vi "DeviceTestPanelGetTimeSeriesRequest_Create.vi"(7 "Header":T2, 8 "error in (no error)":errorcluster, 9 "DeviceTestPanelGetTimeSeriesRequest":T1, 10 "SendTo":string, 11 "ReplyTo":string) -> (0 "error out":errorcluster, 3 "Message":T4)   [LabVIEW 2017]
uses:
  <vilib>/addons/InsightCM/MessageBus/Base/controls/Message.ctl
  <vilib>/addons/InsightCM/MessageBus/Base/controls/MessageHeader.ctl
  <vilib>/addons/InsightCM/MessageBus/Base/controls/KeyValuePair.ctl
  <vilib>/addons/InsightCM/MessageBus/MessageLibrary/Device/controls/DeviceTestPanelGetTimeSeriesRequestBody.ctl
  <vilib>/addons/InsightCM/MessageBus/Base/controls/MessageClassType.ctl
  <vilib>/addons/InsightCM/Utilities/PropertyHelpers/PropertyHelpers.lvlib
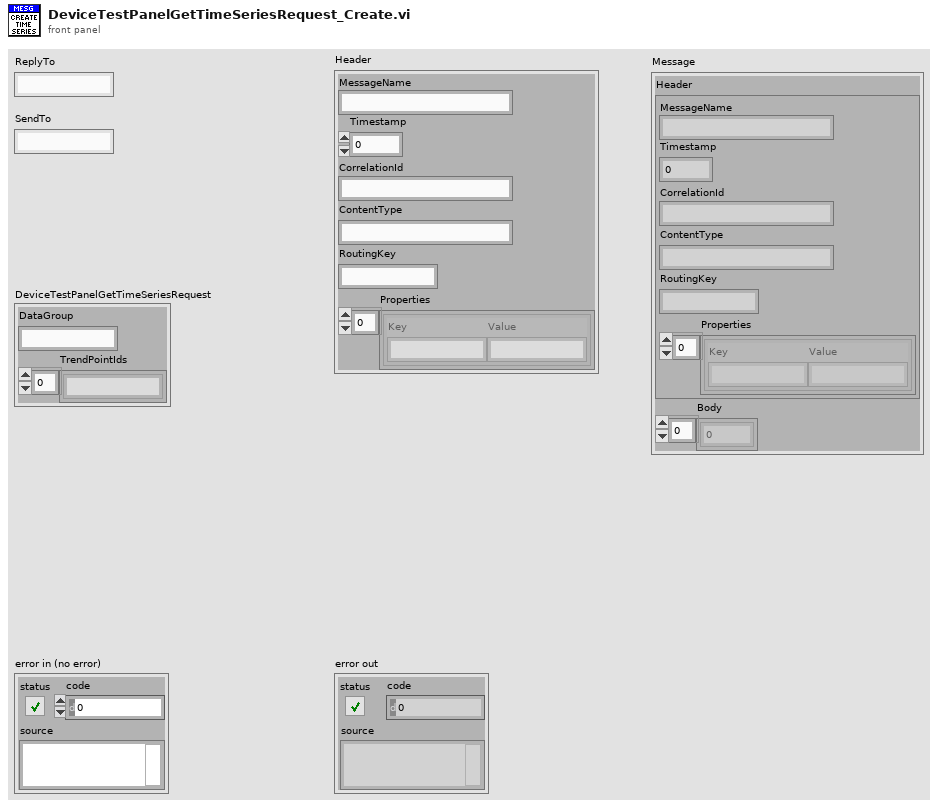
[diagram p1: front panel]
types:
  T1 = typedef "DeviceTestPanelGetTimeSeriesRequestBody.ctl" = cluster{"DataGroup":string, "TrendPointIds":string[]}
  T2 = typedef "MessageHeader.ctl" = cluster{"MessageName":string, "Timestamp":i64, "CorrelationId":string, "ContentType":string, "RoutingKey":string, "Properties":T3[]}
  T3 = typedef "KeyValuePair.ctl" = cluster{"Key":string, "Value":string}
  T4 = typedef "Message.ctl" = cluster{"Header":T2, "Body":u8[]}
  T5 = typedef "MessageClassType.ctl" = enum16{"Request", "Response", "Broadcast", "RoutedMessage"}
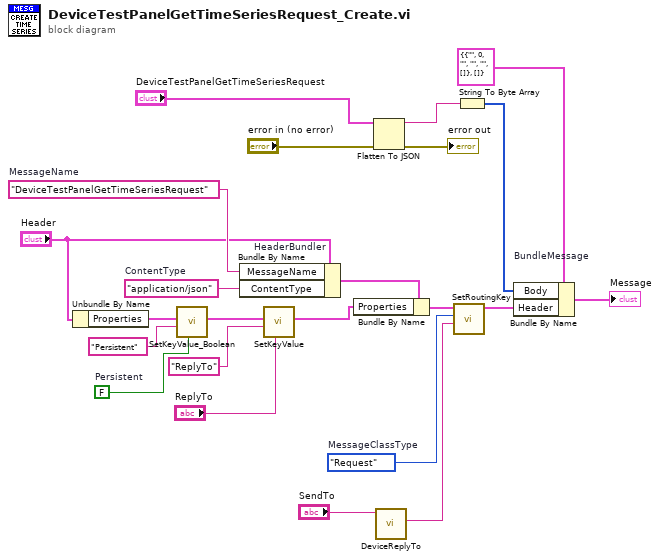
[diagram p0: block diagram]
diagram:
  w19 = MessageClassType."Request"  # MessageClassType
  w14 = FALSE  # Persistent
  w20 = "DeviceTestPanelGetTimeSeriesRequest"  # MessageName
  w17 = "application/json"  # ContentType
  n1 = Unbundle By Name("Header") -> ("Properties"=w16:T3[])
  n2 = call <vilib>:"SetKeyValue_Boolean.vi"("value"=w14, "key"="Persistent" ("Key"), "key value pairs"=w16) -> ("key value pairs out"=w12:T3[])  [unwired: 8 in]
  n3 = Bundle By Name "HeaderBundler"(cluster="Header", "MessageName"=w20, "ContentType"=w17) -> (w10:T2)
  n4 = call <vilib>:"SetKeyValue.vi"("value"="ReplyTo", "key"="ReplyTo" ("Key"), "key value pairs"=w12) -> ("key value pairs out"=w9:T3[])  [unwired: 8 in]
  n5 = Bundle By Name(cluster=w10, "Properties"=w9) -> (w11:T2)
  n6 = Flatten To JSON(anything="DeviceTestPanelGetTimeSeriesRequest", error in (no error)="error in (no error)") -> (JSON string=w2:string, 11:→"error out":errorcluster)  [unwired: 1 in]
  n7 = call <vilib>:"DeviceReplyTo.vi"("Device"="SendTo") -> ("ReplyTo"=w3:string)  [unwired: 10 in]
  n8 = call <vilib>:"SetRoutingKey.vi"("SendTo"=w3, "MessageClassType"=w19, "Message Header in"=w11) -> ("Message Header out"=w13:T2)  [unwired: 8 in]
  n9 = String To Byte Array(string=w2) -> (unsigned byte array=w22:u8[])
  n10 = Bundle By Name "BundleMessage"(cluster=T4 {"Header"={"MessageName"="", "Timestamp"=0, "CorrelationId"="", "ContentType"="", "RoutingKey"="", "Properties"=[]}, "Body"=[]} ("Message"), "Body"=w22, "Header"=w13) -> (→"Message":T4)
